vi "SMU Switch Handshaking - Debug.vi"(8 "error in":errorcluster, 11 "file path (use dialog)":path=path "/home/lvuser/jsontestfile.json") -> (0 "error out":errorcluster)   [LabVIEW 2019]
uses:
  labview-grpc-query-server/VIs/MeasurementServer_FourProbeRawData.ctl
  labview-grpc-query-server/VIs/MeasurementServer_ErrorOutData.ctl
  JSONCluster.ctl
  <instrlib>/niDCPower/nidcpower.llb/niDCPower Send Software Edge Trigger - Signal.ctl
  <instrlib>/niDCPower/nidcpower.llb/niDCPower Configure Software Edge Start Trigger.vi
  <instrlib>/niDCPower/nidcpower.llb/niDCPower Configure Software Edge Sequence Advance Trigger.vi
  SupportVIs.lvlib
  labview-grpc-query-server/VIs/labview-grpc-measurement-server.lvlib
panel:
  in  "Override Channel":bool=TRUE
  in  "Select Next Channel":i32=39
  out "Channels Connected":string[](array[string])=["[ab0->card2r0->c78]", "[ab1->card2r1->c79]", "[ab2->card2r2->c79]", "[ab3->card2r3->c78]"]
  in  "Override Settings":T1={"SMUResourceName"="SMU", "SMUChannels"="0", "SMUSourceMode"=1021, "SMUOutputFunction"=1007, "SMUSourceTransientResponse"=1038, "SMUCurrent"=1.0, "SMUCurrentLevelRange"=1.0, "SMUMeasurementSense"=1008, "SMUMeasurementApertureTime"=0.01, "SMUSourceAdvancedSourceDelay"=0.0001, "SMUVoltage"=6.0, "SMUSourceAdvancedSequenceLoopCount"=127, "SMUMeasurementAdvancedDCNoiseRejection"=1044, "SMUSequenceName"="MySequence", "SMUStep1_Source_DCCurrent_CurrentLevel"=1150009, "SMUStep2_Measurement_ApertureTime"=1150058, "SMUStep3_Source_Advanced_SourceDelay"=1150051, "SMUSequenceNumberOfSteps"=3, "ScanList"="ch0;ch1;ch2;ch3;ch4;ch5;ch6;ch7;ch8;ch9;ch10;ch11;ch12;ch13;ch14;ch15;ch16;ch17;ch18;ch19;ch20;ch21;ch22;ch23;ch24;ch25;ch26;ch27;ch28;ch29;ch30;ch31;ch32;ch33;ch34;ch35;ch36;ch37;ch38;ch39;ch40;ch41;ch42;ch43;ch44;ch45;ch46;ch47;ch48;ch49;ch50;ch51;ch52;ch53;ch54;ch55;ch56;ch57;ch58;ch59;ch60;ch61;ch62;ch63;ch64;ch65;ch66;ch67;ch68;ch69;ch70;ch71;ch72;ch73;ch74;ch75;ch76;ch77;ch78;ch79;ch80;ch81;ch82;ch83;ch84;ch85;ch86;ch87;ch88;ch89;ch90;ch91;ch92;ch93;ch94;ch95;ch96;ch97;ch98;ch99;ch100;ch101;ch102;ch103;ch104;ch105;ch106;ch107;ch108;ch109;ch110;ch111;ch112;ch113;ch114;ch115;ch116;ch117;ch118;ch119;ch120;ch121;ch122;ch123;ch124;ch125;ch126", "Switch1ResourceName"="2526_1", "Switch1Topology"="2526/2-Wire 79x1 Mux", "Switch1ScanList"="ch70:76->com", "Switch2ResourceName"="SwitchBlock1Dev1", "Switch2Topology"="Configured Topology", "Switch2ScanList"="[c2->card1r2->c26], [c3->card1r3->c27]; [c6->card1r2->c26], [c7->card1r3->c27]; [c10->card1r2->c26], [c11->card1r3->c27]; [c14->card1r2->c26], [c15->card1r3->c27]; [c18->card1r2->c26], [c19->card1r3->c27]; [c22->card1r2->c26], [c23->card1r3->c27]; [c30->card1r2->c26], [c31->card1r3->c27];", "DMMResourceName"="DMM", "DMMFunction"=0, "DMMResolution"=0.1, "DMMRange"=10.0, "DMMSampleCount"=0, "DMMApertureTimeUnit"=0, "DMMApertureTime"=0.01, "DMMNumberOfAverages"=1, "DMMAutoZero"=0, "DMMADCCalibration"=0, "DMMSettleTime"=0.0001, "DMMControlAction"=0, "DMMVoltageFaultUpperLimit"=0.0006, "ApplicationNumberOfWeldChannels"=127} {"DMMVoltageFaultUpperLimit" format="%#_6p"}
  in  "Override Settings?":bool=TRUE
  out "Configured Settings":T1={"SMUResourceName"="SMU", "SMUChannels"="0", "SMUSourceMode"=1021, "SMUOutputFunction"=1007, "SMUSourceTransientResponse"=1038, "SMUCurrent"=1.0, "SMUCurrentLevelRange"=1.0, "SMUMeasurementSense"=1008, "SMUMeasurementApertureTime"=0.01, "SMUSourceAdvancedSourceDelay"=0.0001, "SMUVoltage"=6.0, "SMUSourceAdvancedSequenceLoopCount"=127, "SMUMeasurementAdvancedDCNoiseRejection"=1044, "SMUSequenceName"="MySequence", "SMUStep1_Source_DCCurrent_CurrentLevel"=1150009, "SMUStep2_Measurement_ApertureTime"=1150058, "SMUStep3_Source_Advanced_SourceDelay"=1150051, "SMUSequenceNumberOfSteps"=3, "ScanList"="ch0;ch1;ch2;ch3;ch4;ch5;ch6;ch7;ch8;ch9;ch10;ch11;ch12;ch13;ch14;ch15;ch16;ch17;ch18;ch19;ch20;ch21;ch22;ch23;ch24;ch25;ch26;ch27;ch28;ch29;ch30;ch31;ch32;ch33;ch34;ch35;ch36;ch37;ch38;ch39;ch40;ch41;ch42;ch43;ch44;ch45;ch46;ch47;ch48;ch49;ch50;ch51;ch52;ch53;ch54;ch55;ch56;ch57;ch58;ch59;ch60;ch61;ch62;ch63;ch64;ch65;ch66;ch67;ch68;ch69;ch70;ch71;ch72;ch73;ch74;ch75;ch76;ch77;ch78;ch79;ch80;ch81;ch82;ch83;ch84;ch85;ch86;ch87;ch88;ch89;ch90;ch91;ch92;ch93;ch94;ch95;ch96;ch97;ch98;ch99;ch100;ch101;ch102;ch103;ch104;ch105;ch106;ch107;ch108;ch109;ch110;ch111;ch112;ch113;ch114;ch115;ch116;ch117;ch118;ch119;ch120;ch121;ch122;ch123;ch124;ch125;ch126", "Switch1ResourceName"="2526_1", "Switch1Topology"="2526/2-Wire 79x1 Mux", "Switch1ScanList"="ch70:76->com", "Switch2ResourceName"="SwitchBlock1Dev1", "Switch2Topology"="Configured Topology", "Switch2ScanList"="[c2->card1r2->c26], [c3->card1r3->c27]; [c6->card1r2->c26], [c7->card1r3->c27]; [c10->card1r2->c26], [c11->card1r3->c27]; [c14->card1r2->c26], [c15->card1r3->c27]; [c18->card1r2->c26], [c19->card1r3->c27]; [c22->card1r2->c26], [c23->card1r3->c27]; [c30->card1r2->c26], [c31->card1r3->c27];", "DMMResourceName"="DMM", "DMMFunction"=0, "DMMResolution"=0.1, "DMMRange"=10.0, "DMMSampleCount"=0, "DMMApertureTimeUnit"=0, "DMMApertureTime"=0.01, "DMMNumberOfAverages"=1, "DMMAutoZero"=0, "DMMADCCalibration"=0, "DMMSettleTime"=0.0001, "DMMControlAction"=0, "DMMVoltageFaultUpperLimit"=0.0006, "ApplicationNumberOfWeldChannels"=127} {"DMMVoltageFaultUpperLimit" format="%#_6p"}
  out "All Results":T2[](array[typedef])=[{"Positive Voltage"=0.4227098432914551, "Positive Current"=-8.493421060188494e-06, "Negative Voltage"=0.06989759298606142, "Negative Current"=-7.73956711993401e-06, "Impedance"=-468011.41635777906, "ErrorOutData"={"ErrorCode"=-3, "ErrorMessage"="SMU HI or LO lead disconnected\n- SMU in compliance\n- SMU Fault = True\rDMM HI SENSE or LO SENSE lead disconnected\n- DMM measures NaN, or \n- DMM overrange warning, or\n- DMM voltage > 50uV "}}, {"Positive Voltage"=0.00044270637570739045, "Positive Current"=0.9998336100314509, "Negative Voltage"=-0.0005552929370042879, "Negative Current"=-0.9996807598629482, "Impedance"=0.0004991208504114857, "ErrorOutData"={"ErrorCode"=0, "ErrorMessage"="\r"}}, {"Positive Voltage"=0.0004435264921852196, "Positive Current"=0.9998415883189853, "Negative Voltage"=-0.0005563935478104583, "Negative Current"=-0.9996805713994632, "Impedance"=0.000500079499062154, "ErrorOutData"={"ErrorCode"=0, "ErrorMessage"="\r"}}, {"Positive Voltage"=0.0004431847687781547, "Positive Current"=0.9998360600567567, "Negative Voltage"=-0.0005561418564061973, "Negative Current"=-0.999680791273529, "Impedance"=0.000499784047591045, "ErrorOutData"={"ErrorCode"=0, "ErrorMessage"="\r"}}, {"Positive Voltage"=0.0004426508664081714, "Positive Current"=0.9998373793011521, "Negative Voltage"=-0.0005564300544965975, "Negative Current"=-0.9996810739687567, "Impedance"=0.0004996607654562646, "ErrorOutData"={"ErrorCode"=0, "ErrorMessage"="\r"}}, {"Positive Voltage"=0.000442879495774044, "Positive Current"=0.9998407088227216, "Negative Voltage"=-0.0005564269589209733, "Negative Current"=-0.9996801630619121, "Impedance"=0.0004997729549845249, "ErrorOutData"={"ErrorCode"=0, "ErrorMessage"="\r"}}, {"Positive Voltage"=0.0004429170648054572, "Positive Current"=0.9998418396036319, "Negative Voltage"=-0.0005554367475981239, "Negative Current"=-0.9996802572936547, "Impedance"=0.0004992962138066661, "ErrorOutData"={"ErrorCode"=0, "ErrorMessage"="\r"}}, {"Positive Voltage"=0.0004437757493413744, "Positive Current"=0.9998415569084044, "Negative Voltage"=-0.0005568618872958528, "Negative Current"=-0.9996772418778936, "Impedance"=0.0005004392242996721, "ErrorOutData"={"ErrorCode"=0, "ErrorMessage"="\r"}}, {"Positive Voltage"=0.0004425981290562125, "Positive Current"=0.9998418710142127, "Negative Voltage"=-0.0005563588351510922, "Negative Current"=-0.9996784354799657, "Impedance"=0.0004995983091358584, "ErrorOutData"={"ErrorCode"=0, "ErrorMessage"="\r"}}, {"Positive Voltage"=0.0004431512451012525, "Positive Current"=0.999839829326458, "Negative Voltage"=-0.0005559987986000694, "Negative Current"=-0.9996786867646126, "Impedance"=0.0004996953194785092, "ErrorOutData"={"ErrorCode"=0, "ErrorMessage"="\r"}}, {"Positive Voltage"=0.0004428252458112706, "Positive Current"=0.9998417767824702, "Negative Voltage"=-0.0005563071531090114, "Negative Current"=-0.9996822361602478, "Impedance"=0.0004996851212853651, "ErrorOutData"={"ErrorCode"=0, "ErrorMessage"="\r"}}, {"Positive Voltage"=0.0004432269671022045, "Positive Current"=0.9998400177899429, "Negative Voltage"=-0.0005555003827833456, "Negative Current"=-0.9996774931625403, "Impedance"=0.0004994841727641584, "ErrorOutData"={"ErrorCode"=0, "ErrorMessage"="\r"}}, {"Positive Voltage"=0.00044334477486081486, "Positive Current"=0.9998417453718894, "Negative Voltage"=-0.0005564183194508279, "Negative Current"=-0.9996779329106722, "Impedance"=0.0005000016279761572, "ErrorOutData"={"ErrorCode"=0, "ErrorMessage"="\r"}}, {"Positive Voltage"=0.0004424807152799528, "Positive Current"=0.9998395466312303, "Negative Voltage"=-0.0005557886160507434, "Negative Current"=-0.9996787181751934, "Impedance"=0.0004992549199981127, "ErrorOutData"={"ErrorCode"=0, "ErrorMessage"="\r"}}, {"Positive Voltage"=0.00044335168362277214, "Positive Current"=0.9998386043138051, "Negative Voltage"=-0.0005557412185667331, "Negative Current"=-0.9996809797370141, "Impedance"=0.0004996664749666751, "ErrorOutData"={"ErrorCode"=0, "ErrorMessage"="\r"}}, {"Positive Voltage"=0.00044343080372150783, "Positive Current"=0.9998369395530203, "Negative Voltage"=-0.0005562687679712933, "Negative Current"=-0.9996811996110799, "Impedance"=0.0004999702438862225, "ErrorOutData"={"ErrorCode"=0, "ErrorMessage"="\r"}}, {"Positive Voltage"=0.0004416126595923773, "Positive Current"=0.9998378504598648, "Negative Voltage"=-0.0005565125515869184, "Negative Current"=-0.999679000870421, "Impedance"=0.0004991831954380576, "ErrorOutData"={"ErrorCode"=0, "ErrorMessage"="\r"}}, {"Positive Voltage"=0.0004425058457256834, "Positive Current"=0.9998383530291582, "Negative Voltage"=-0.0005561486666725616, "Negative Current"=-0.9996688552528084, "Impedance"=0.0004994503186894321, "ErrorOutData"={"ErrorCode"=0, "ErrorMessage"="\r"}}, {"Positive Voltage"=0.00044199289477433746, "Positive Current"=0.9998407402333024, "Negative Voltage"=-0.0005564866613180825, "Negative Current"=-0.9996799117772655, "Impedance"=0.0004993594615231526, "ErrorOutData"={"ErrorCode"=0, "ErrorMessage"="\r"}}, {"Positive Voltage"=0.00044318225010526666, "Positive Current"=0.9998403318957514, "Negative Voltage"=-0.0005570190932896488, "Negative Current"=-0.9996808855052717, "Impedance"=0.0005002204201138594, "ErrorOutData"={"ErrorCode"=0, "ErrorMessage"="\r"}}, {"Positive Voltage"=0.0004425723091413646, "Positive Current"=0.9998389184196134, "Negative Voltage"=-0.0005564301952045792, "Negative Current"=-0.9996751059583964, "Impedance"=0.0004996226543880852, "ErrorOutData"={"ErrorCode"=0, "ErrorMessage"="\r"}}, {"Positive Voltage"=0.0004422648410927191, "Positive Current"=0.9998419966565362, "Negative Voltage"=-0.0005559992699718129, "Negative Current"=-0.9996819220544393, "Impedance"=0.0004992508975376892, "ErrorOutData"={"ErrorCode"=0, "ErrorMessage"="\r"}}, {"Positive Voltage"=0.00044284054076900033, "Positive Current"=0.9998383530291582, "Negative Voltage"=-0.0005559332357154717, "Negative Current"=-0.9996781213741572, "Impedance"=0.0004995076506096407, "ErrorOutData"={"ErrorCode"=0, "ErrorMessage"="\r"}}, {"Positive Voltage"=0.00044220070639415055, "Positive Current"=0.9998387613667092, "Negative Voltage"=-0.0005564631279079567, "Negative Current"=-0.9996743835150368, "Impedance"=0.0004994534978969441, "ErrorOutData"={"ErrorCode"=0, "ErrorMessage"="\r"}}, {"Positive Voltage"=0.0004425694386985146, "Positive Current"=0.9998407402333024, "Negative Voltage"=-0.0005558320103926432, "Negative Current"=-0.9996787181751934, "Impedance"=0.0004993206967267169, "ErrorOutData"={"ErrorCode"=0, "ErrorMessage"="\r"}}, {"Positive Voltage"=0.00044327916976382933, "Positive Current"=0.9998404575380748, "Negative Voltage"=-0.0005567623363980099, "Negative Current"=-0.9996809169158525, "Impedance"=0.00050014044307726, "ErrorOutData"={"ErrorCode"=0, "ErrorMessage"="\r"}}, {"Positive Voltage"=0.000442306385124646, "Positive Current"=0.9998411171602725, "Negative Voltage"=-0.0005558222241524345, "Negative Current"=-0.9996798803666846, "Impedance"=0.0004991838597902116, "ErrorOutData"={"ErrorCode"=0, "ErrorMessage"="\r"}}, {"Positive Voltage"=0.00044307567787908264, "Positive Current"=0.9998385729032242, "Negative Voltage"=-0.0005561501018939907, "Negative Current"=-0.9996810425581757, "Impedance"=0.0004997329218710848, "ErrorOutData"={"ErrorCode"=0, "ErrorMessage"="\r"}}, {"Positive Voltage"=0.0004419110308699325, "Positive Current"=0.9998370651953438, "Negative Voltage"=-0.0005568956923887257, "Negative Current"=-0.9996802887042355, "Impedance"=0.0004995239082625241, "ErrorOutData"={"ErrorCode"=0, "ErrorMessage"="\r"}}, {"Positive Voltage"=0.00044257959781487293, "Positive Current"=0.9998401434322665, "Negative Voltage"=-0.0005564586393233032, "Negative Current"=-0.9996774303413787, "Impedance"=0.0004996396382016856, "ErrorOutData"={"ErrorCode"=0, "ErrorMessage"="\r"}}, {"Positive Voltage"=0.00044266013906423565, "Positive Current"=0.9998405203592365, "Negative Voltage"=-0.0005567629766193307, "Negative Current"=-0.9996879842965423, "Impedance"=0.0004998293914572717, "ErrorOutData"={"ErrorCode"=0, "ErrorMessage"="\r"}}, {"Positive Voltage"=0.0004422246267512286, "Positive Current"=0.9998426876893148, "Negative Voltage"=-0.0005563399873167974, "Negative Current"=-0.9996818906438585, "Impedance"=0.0004994010200667005, "ErrorOutData"={"ErrorCode"=0, "ErrorMessage"="\r"}}, {"Positive Voltage"=0.00044222253723768596, "Positive Current"=0.9998389184196134, "Negative Voltage"=-0.0005559288456264137, "Negative Current"=-0.9996776188048637, "Impedance"=0.0004991963628616098, "ErrorOutData"={"ErrorCode"=0, "ErrorMessage"="\r"}}, {"Positive Voltage"=0.00044335341433095643, "Positive Current"=0.9998379761021882, "Negative Voltage"=-0.0005566963584248685, "Negative Current"=-0.999682581676637, "Impedance"=0.0005001447816404218, "ErrorOutData"={"ErrorCode"=0, "ErrorMessage"="\r"}}, {"Positive Voltage"=0.00044284327753927097, "Positive Current"=0.999840426127494, "Negative Voltage"=-0.0005560568476783757, "Negative Current"=-0.9996789066386784, "Impedance"=0.000499570126104132, "ErrorOutData"={"ErrorCode"=0, "ErrorMessage"="\r"}}, {"Positive Voltage"=0.00044303544946679564, "Positive Current"=0.9998377562281222, "Negative Voltage"=-0.0005555104504395151, "Negative Current"=-0.9996565737156984, "Impedance"=0.0004993992155678514, "ErrorOutData"={"ErrorCode"=0, "ErrorMessage"="\r"}}, {"Positive Voltage"=0.0004430247275185058, "Positive Current"=0.9998403004851706, "Negative Voltage"=-0.0005556892058608842, "Negative Current"=-0.9996790636915827, "Impedance"=0.000499476999959229, "ErrorOutData"={"ErrorCode"=0, "ErrorMessage"="\r"}}, {"Positive Voltage"=0.0004431882231591376, "Positive Current"=0.9998384786714817, "Negative Voltage"=-0.0005559463074870784, "Negative Current"=-0.9996799745984271, "Impedance"=0.0004996875767824414, "ErrorOutData"={"ErrorCode"=0, "ErrorMessage"="\r"}}, {"Positive Voltage"=0.0004431953218768679, "Positive Current"=0.9998368767318586, "Negative Voltage"=-0.0005563412396178422, "Negative Current"=-0.9996809797370141, "Impedance"=0.0004998887898205026, "ErrorOutData"={"ErrorCode"=0, "ErrorMessage"="\r"}}, {"Positive Voltage"=0.00044275691801481633, "Positive Current"=0.9998376934069605, "Negative Voltage"=-0.0005565454420779015, "Negative Current"=-0.9996735982505158, "Impedance"=0.0004997733017373237, "ErrorOutData"={"ErrorCode"=0, "ErrorMessage"="\r"}}, {"Positive Voltage"=0.00044314802288844546, "Positive Current"=0.9998382902079966, "Negative Voltage"=-0.0005562527554028524, "Negative Current"=-0.9996796919031994, "Impedance"=0.0004998208504412039, "ErrorOutData"={"ErrorCode"=0, "ErrorMessage"="\r"}}, {"Positive Voltage"=0.0004420522031890927, "Positive Current"=0.9998410229285299, "Negative Voltage"=-0.0005573198777091121, "Negative Current"=-0.9996810111475949, "Impedance"=0.0004998054854444067, "ErrorOutData"={"ErrorCode"=0, "ErrorMessage"="\r"}}, {"Positive Voltage"=0.00044142678434708, "Positive Current"=0.9998407716438832, "Negative Voltage"=-0.0005555250137157432, "Negative Current"=-0.9996751373689772, "Impedance"=0.0004985965820872151, "ErrorOutData"={"ErrorCode"=0, "ErrorMessage"="\r"}}, {"Positive Voltage"=0.000443285860428411, "Positive Current"=0.9998395466312303, "Negative Voltage"=-0.0005562909083723878, "Negative Current"=-0.9996787181751934, "Impedance"=0.0004999087962307609, "ErrorOutData"={"ErrorCode"=0, "ErrorMessage"="\r"}}, {"Positive Voltage"=0.0004429727148126581, "Positive Current"=0.9998380389233499, "Negative Voltage"=-0.0005558561207054957, "Negative Current"=-0.9996800688301695, "Impedance"=0.000499534778727435, "ErrorOutData"={"ErrorCode"=0, "ErrorMessage"="\r"}}, {"Positive Voltage"=0.00044351776829028403, "Positive Current"=0.9998382902079966, "Negative Voltage"=-0.0005558105664960561, "Negative Current"=-0.9996829271930263, "Impedance"=0.0004997838112892179, "ErrorOutData"={"ErrorCode"=0, "ErrorMessage"="\r"}}, {"Positive Voltage"=0.00044180997439667607, "Positive Current"=0.9998401120216855, "Negative Voltage"=-0.000557451756266006, "Negative Current"=-0.9996774303413787, "Impedance"=0.0004997514197758612, "ErrorOutData"={"ErrorCode"=0, "ErrorMessage"="\r"}}, {"Positive Voltage"=0.00044238172017864306, "Positive Current"=0.9998386043138051, "Negative Voltage"=-0.0005569053801333431, "Negative Current"=-0.9996742578727136, "Impedance"=0.0004997652774382456, "ErrorOutData"={"ErrorCode"=0, "ErrorMessage"="\r"}}, {"Positive Voltage"=0.0004427133055755449, "Positive Current"=0.9998418710142127, "Negative Voltage"=-0.0005560911241429957, "Negative Current"=-0.9996782156058999, "Impedance"=0.0004995220785237866, "ErrorOutData"={"ErrorCode"=0, "ErrorMessage"="\r"}}, {"Positive Voltage"=0.0004414873591336821, "Positive Current"=0.9998379446916074, "Negative Voltage"=-0.0005556362926239444, "Negative Current"=-0.9996797547243612, "Impedance"=0.000498682083208802, "ErrorOutData"={"ErrorCode"=0, "ErrorMessage"="\r"}}, {"Positive Voltage"=0.0004430884963763173, "Positive Current"=0.999840426127494, "Negative Voltage"=-0.0005560188072752255, "Negative Current"=-0.9996811996110799, "Impedance"=0.0004996731672169323, "ErrorOutData"={"ErrorCode"=0, "ErrorMessage"="\r"}}, {"Positive Voltage"=0.00044224104033742503, "Positive Current"=0.9998412113920151, "Negative Voltage"=-0.0005563428929366435, "Negative Current"=-0.9996808540946909, "Impedance"=0.0004994113095876249, "ErrorOutData"={"ErrorCode"=0, "ErrorMessage"="\r"}}, {"Positive Voltage"=0.0004429970643290835, "Positive Current"=0.9998384786714817, "Negative Voltage"=-0.000556510075126418, "Negative Current"=-0.9996776502154447, "Impedance"=0.0004998745071448354, "ErrorOutData"={"ErrorCode"=0, "ErrorMessage"="\r"}}, {"Positive Voltage"=0.00044266864486179787, "Positive Current"=0.9998386043138051, "Negative Voltage"=-0.0005569831564708411, "Negative Current"=-0.9996800374195887, "Impedance"=0.000499946227291002, "ErrorOutData"={"ErrorCode"=0, "ErrorMessage"="\r"}}, {"Positive Voltage"=0.0004427809439028817, "Positive Current"=0.9998398607370388, "Negative Voltage"=-0.0005559008939856245, "Negative Current"=-0.9996806970417864, "Impedance"=0.0004994606502060152, "ErrorOutData"={"ErrorCode"=0, "ErrorMessage"="\r"}}, {"Positive Voltage"=0.00044351095098851617, "Positive Current"=0.9998402690745898, "Negative Voltage"=-0.0005555750424390234, "Negative Current"=-0.9996839637421944, "Impedance"=0.0004996618580711573, "ErrorOutData"={"ErrorCode"=0, "ErrorMessage"="\r"}}, {"Positive Voltage"=0.0004428245211651586, "Positive Current"=0.9998405203592365, "Negative Voltage"=-0.0005560609563514788, "Negative Current"=-0.9996781841953188, "Impedance"=0.0004995629574463847, "ErrorOutData"={"ErrorCode"=0, "ErrorMessage"="\r"}}, {"Positive Voltage"=0.00044282480961652413, "Positive Current"=0.9998400806111047, "Negative Voltage"=-0.000555894519914007, "Negative Current"=-0.9996828957824455, "Impedance"=0.0004994787963536564, "ErrorOutData"={"ErrorCode"=0, "ErrorMessage"="\r"}}, {"Positive Voltage"=0.00044260601573864906, "Positive Current"=0.9998393267571645, "Negative Voltage"=-0.000556537344333492, "Negative Current"=-0.9996795034397143, "Impedance"=0.0004996918983622485, "ErrorOutData"={"ErrorCode"=0, "ErrorMessage"="\r"}}, {"Positive Voltage"=0.00044254660179290423, "Positive Current"=0.9998405831803983, "Negative Voltage"=-0.000556063974537708, "Negative Current"=-0.9996802572936547, "Impedance"=0.00049942494027412, "ErrorOutData"={"ErrorCode"=0, "ErrorMessage"="\r"}}, {"Positive Voltage"=0.00044281629678356534, "Positive Current"=0.9998393267571645, "Negative Voltage"=-0.0005562237976999881, "Negative Current"=-0.9996801002407505, "Impedance"=0.0004996401040141508, "ErrorOutData"={"ErrorCode"=0, "ErrorMessage"="\r"}}, {"Positive Voltage"=0.0004432513095832306, "Positive Current"=0.9998374421223138, "Negative Voltage"=-0.0005564357039221052, "Negative Current"=-0.9996799117772655, "Impedance"=0.0004999641596286653, "ErrorOutData"={"ErrorCode"=0, "ErrorMessage"="\r"}}, {"Positive Voltage"=0.00044258595078029803, "Positive Current"=0.9998409286967875, "Negative Voltage"=-0.0005558095111861886, "Negative Current"=-0.9996796604926186, "Impedance"=0.0004993174200677926, "ErrorOutData"={"ErrorCode"=0, "ErrorMessage"="\r"}}, {"Positive Voltage"=0.00044370010472981504, "Positive Current"=0.9998396408629728, "Negative Voltage"=-0.0005551230180442423, "Negative Current"=-0.9996802258830739, "Impedance"=0.0004995314822250351, "ErrorOutData"={"ErrorCode"=0, "ErrorMessage"="\r"}}, {"Positive Voltage"=0.0004421424532892677, "Positive Current"=0.9998386043138051, "Negative Voltage"=-0.0005560646288298306, "Negative Current"=-0.9996828957824455, "Impedance"=0.0004992229801335208, "ErrorOutData"={"ErrorCode"=0, "ErrorMessage"="\r"}}, {"Positive Voltage"=0.0004429717157859826, "Positive Current"=0.9998399549687813, "Negative Voltage"=-0.000554845260486166, "Negative Current"=-0.9996752630113004, "Impedance"=0.0004990294483880684, "ErrorOutData"={"ErrorCode"=0, "ErrorMessage"="\r"}}, {"Positive Voltage"=0.0004434583543445421, "Positive Current"=0.9998400806111047, "Negative Voltage"=-0.0005564016807318582, "Negative Current"=-0.9996788124069358, "Impedance"=0.0005000503063850666, "ErrorOutData"={"ErrorCode"=0, "ErrorMessage"="\r"}}, {"Positive Voltage"=0.00044290748259182754, "Positive Current"=0.9998385100820625, "Negative Voltage"=-0.0005550344001566628, "Negative Current"=-0.9996828015507031, "Impedance"=0.0004990903957575691, "ErrorOutData"={"ErrorCode"=0, "ErrorMessage"="\r"}}, {"Positive Voltage"=0.00044336150503997346, "Positive Current"=0.9998409601073683, "Negative Voltage"=-0.000556003906299844, "Negative Current"=-0.9996812310216607, "Impedance"=0.0004998021106109987, "ErrorOutData"={"ErrorCode"=0, "ErrorMessage"="\r"}}, {"Positive Voltage"=0.00044301018534848176, "Positive Current"=0.9998403318957514, "Negative Voltage"=-0.0005556932371445914, "Negative Current"=-0.9996803829359779, "Impedance"=0.0004994714058649398, "ErrorOutData"={"ErrorCode"=0, "ErrorMessage"="\r"}}, {"Positive Voltage"=0.0004430160036235707, "Positive Current"=0.99983841585032, "Negative Voltage"=-0.0005551907900441595, "Negative Current"=-0.9996821733390862, "Impedance"=0.0004992230633005871, "ErrorOutData"={"ErrorCode"=0, "ErrorMessage"="\r"}}, {"Positive Voltage"=0.00044397347923422236, "Positive Current"=0.9998403004851706, "Negative Voltage"=-0.0005554320690576878, "Negative Current"=-0.9996791265127443, "Impedance"=0.0004998228748356905, "ErrorOutData"={"ErrorCode"=0, "ErrorMessage"="\r"}}, {"Positive Voltage"=0.0004427937975771129, "Positive Current"=0.9998398607370388, "Negative Voltage"=-0.0005560462101548804, "Negative Current"=-0.9996791893339061, "Impedance"=0.0004995401307612215, "ErrorOutData"={"ErrorCode"=0, "ErrorMessage"="\r"}}, {"Positive Voltage"=0.0004433314005670486, "Positive Current"=0.9998418081930511, "Negative Voltage"=-0.0005552790772679779, "Negative Current"=-0.9996795348502954, "Impedance"=0.0004994247654866759, "ErrorOutData"={"ErrorCode"=0, "ErrorMessage"="\r"}}, {"Positive Voltage"=0.00044341707062238586, "Positive Current"=0.9998393581677453, "Negative Voltage"=-0.0005556148205857652, "Negative Current"=-0.9996809797370141, "Impedance"=0.0004996357737751287, "ErrorOutData"={"ErrorCode"=0, "ErrorMessage"="\r"}}, {"Positive Voltage"=0.0004425868794529835, "Positive Current"=0.9998395780418111, "Negative Voltage"=-0.0005556132587271592, "Negative Current"=-0.9996740065880667, "Impedance"=0.0004992214835914284, "ErrorOutData"={"ErrorCode"=0, "ErrorMessage"="\r"}}, {"Positive Voltage"=0.0004435337456817334, "Positive Current"=0.9998420280671171, "Negative Voltage"=-0.0005550171001101737, "Negative Current"=-0.9996788124069358, "Impedance"=0.0004993950678479388, "ErrorOutData"={"ErrorCode"=0, "ErrorMessage"="\r"}}, {"Positive Voltage"=0.0004429351035688524, "Positive Current"=0.9998386357243859, "Negative Voltage"=-0.000554562233414135, "Negative Current"=-0.9996781841953188, "Impedance"=0.0004988691903192113, "ErrorOutData"={"ErrorCode"=0, "ErrorMessage"="\r"}}, {"Positive Voltage"=0.0004439495518417443, "Positive Current"=0.9998382273868349, "Negative Voltage"=-0.0005553659996243591, "Negative Current"=-0.9996779015000914, "Impedance"=0.0004997786899685545, "ErrorOutData"={"ErrorCode"=0, "ErrorMessage"="\r"}}, {"Positive Voltage"=0.00044354244847046975, "Positive Current"=0.9998349606864272, "Negative Voltage"=-0.0005560542656868961, "Negative Current"=-0.999678152784738, "Impedance"=0.0004999200592498544, "ErrorOutData"={"ErrorCode"=0, "ErrorMessage"="\r"}}, {"Positive Voltage"=0.0004426065222873858, "Positive Current"=0.9998414312660809, "Negative Voltage"=-0.0005557233556883142, "Negative Current"=-0.9996766764874385, "Impedance"=0.0004992852398307783, "ErrorOutData"={"ErrorCode"=0, "ErrorMessage"="\r"}}, {"Positive Voltage"=0.00044288011488916983, "Positive Current"=0.9998413684449193, "Negative Voltage"=-0.0005557669892337818, "Negative Current"=-0.999679786134942, "Impedance"=0.0004994431300892072, "ErrorOutData"={"ErrorCode"=0, "ErrorMessage"="\r"}}, {"Positive Voltage"=0.0004428762032072458, "Positive Current"=0.9998377248175414, "Negative Voltage"=-0.0005548895553591558, "Negative Current"=-0.999676959182666, "Impedance"=0.0004990039665876733, "ErrorOutData"={"ErrorCode"=0, "ErrorMessage"="\r"}}, {"Positive Voltage"=0.00044407517592880336, "Positive Current"=0.999837787638703, "Negative Voltage"=-0.0005548592187180599, "Negative Current"=-0.9996804771677206, "Impedance"=0.0004995875317715949, "ErrorOutData"={"ErrorCode"=0, "ErrorMessage"="\r"}}, {"Positive Voltage"=0.000442873438295384, "Positive Current"=0.9998397665052963, "Negative Voltage"=-0.0005559368941230299, "Negative Current"=-0.9996825502660562, "Impedance"=0.0004995244734408377, "ErrorOutData"={"ErrorCode"=0, "ErrorMessage"="\r"}}, {"Positive Voltage"=0.00044300414897601896, "Positive Current"=0.9998385100820625, "Negative Voltage"=-0.0005553567410390924, "Negative Current"=-0.99967859253287, "Impedance"=0.0004993010005813268, "ErrorOutData"={"ErrorCode"=0, "ErrorMessage"="\r"}}, {"Positive Voltage"=0.00044446186960717495, "Positive Current"=0.9998381959762541, "Negative Voltage"=-0.0005549508266502684, "Negative Current"=-0.9996785297117083, "Impedance"=0.0004998271249336918, "ErrorOutData"={"ErrorCode"=0, "ErrorMessage"="\r"}}, {"Positive Voltage"=0.00044342652619882645, "Positive Current"=0.9998413998555001, "Negative Voltage"=-0.0005558535176078165, "Negative Current"=-0.9996788438175166, "Impedance"=0.0004997599033911337, "ErrorOutData"={"ErrorCode"=0, "ErrorMessage"="\r"}}, {"Positive Voltage"=0.0004433281853896422, "Positive Current"=0.9998417139613086, "Negative Voltage"=-0.0005547129879469202, "Negative Current"=-0.9996754200642048, "Impedance"=0.0004991410957940947, "ErrorOutData"={"ErrorCode"=0, "ErrorMessage"="\r"}}, {"Positive Voltage"=0.0004441760213400837, "Positive Current"=0.9998393895783262, "Negative Voltage"=-0.0005557373279910032, "Negative Current"=-0.9996753886536238, "Impedance"=0.0005000779990309699, "ErrorOutData"={"ErrorCode"=0, "ErrorMessage"="\r"}}, {"Positive Voltage"=0.0004441705266933572, "Positive Current"=0.9998400177899429, "Negative Voltage"=-0.0005539599117875031, "Negative Current"=-0.9996783412482233, "Impedance"=0.0004991854333165481, "ErrorOutData"={"ErrorCode"=0, "ErrorMessage"="\r"}}, {"Positive Voltage"=0.0004443011881261959, "Positive Current"=0.9998402690745898, "Negative Voltage"=-0.0005546106721372168, "Negative Current"=-0.9996799745984271, "Impedance"=0.000499575767449327, "ErrorOutData"={"ErrorCode"=0, "ErrorMessage"="\r"}}, {"Positive Voltage"=0.000443970418835595, "Positive Current"=0.9998430646162849, "Negative Voltage"=-0.0005559718600567603, "Negative Current"=-0.9996837124575475, "Impedance"=0.0005000894663464827, "ErrorOutData"={"ErrorCode"=0, "ErrorMessage"="\r"}}, {"Positive Voltage"=0.00044269900964449057, "Positive Current"=0.9998405831803983, "Negative Voltage"=-0.0005546125787303834, "Negative Current"=-0.999673535429354, "Impedance"=0.0004987769674106114, "ErrorOutData"={"ErrorCode"=0, "ErrorMessage"="\r"}}, {"Positive Voltage"=0.00044476273845142405, "Positive Current"=0.999839201114841, "Negative Voltage"=-0.0005547441406943128, "Negative Current"=-0.9996797233137802, "Impedance"=0.0004998736780805183, "ErrorOutData"={"ErrorCode"=0, "ErrorMessage"="\r"}}, {"Positive Voltage"=0.0004437515686745285, "Positive Current"=0.9998401434322665, "Negative Voltage"=-0.0005555780395190644, "Negative Current"=-0.999680791273529, "Impedance"=0.0004997845188055667, "ErrorOutData"={"ErrorCode"=0, "ErrorMessage"="\r"}}, {"Positive Voltage"=0.00044478751712719494, "Positive Current"=0.9998395780418111, "Negative Voltage"=-0.0005546307652371631, "Negative Current"=-0.9996826444977989, "Impedance"=0.0004998285445885109, "ErrorOutData"={"ErrorCode"=0, "ErrorMessage"="\r"}}, {"Positive Voltage"=0.0004436276471540641, "Positive Current"=0.999839829326458, "Negative Voltage"=-0.0005545804621333089, "Negative Current"=-0.9996774617519595, "Impedance"=0.0004992245447144898, "ErrorOutData"={"ErrorCode"=0, "ErrorMessage"="\r"}}, {"Positive Voltage"=0.0004442093198842178, "Positive Current"=0.9998427190998956, "Negative Voltage"=-0.000554744802021834, "Negative Current"=-0.9996790322810019, "Impedance"=0.0004995965266275099, "ErrorOutData"={"ErrorCode"=0, "ErrorMessage"="\r"}}, {"Positive Voltage"=0.00044512598314445673, "Positive Current"=0.9998256945650782, "Negative Voltage"=-0.0005556313889507473, "Negative Current"=-0.9996786867646126, "Impedance"=0.0005005027152927218, "ErrorOutData"={"ErrorCode"=0, "ErrorMessage"="\r"}}, {"Positive Voltage"=0.00044217321205431066, "Positive Current"=0.9998455460521715, "Negative Voltage"=-0.000555220317614351, "Negative Current"=-0.9996705514241739, "Impedance"=0.0004988174543468315, "ErrorOutData"={"ErrorCode"=0, "ErrorMessage"="\r"}}, {"Positive Voltage"=-5.4936250649797755e-05, "Positive Current"=-8.399189317657985e-06, "Negative Voltage"=-5.6232501835270916e-05, "Negative Current"=-7.770977700782139e-06, "Impedance"=-2.0633989417762395, "ErrorOutData"={"ErrorCode"=-1, "ErrorMessage"="SMU HI or LO lead disconnected\n- SMU in compliance\n- SMU Fault = True\r"}}, {"Positive Voltage"=-5.5786872618300966e-05, "Positive Current"=-8.556242221877813e-06, "Negative Voltage"=-5.625998210431502e-05, "Negative Current"=-7.67674595824816e-06, "Impedance"=-0.5379323432956326, "ErrorOutData"={"ErrorCode"=-1, "ErrorMessage"="SMU HI or LO lead disconnected\n- SMU in compliance\n- SMU Fault = True\r"}}, {"Positive Voltage"=-5.679127434122135e-05, "Positive Current"=-8.493421060188494e-06, "Negative Voltage"=-5.500922180968423e-05, "Negative Current"=-7.896620024153839e-06, "Impedance"=2.9860077713297404, "ErrorOutData"={"ErrorCode"=-1, "ErrorMessage"="SMU HI or LO lead disconnected\n- SMU in compliance\n- SMU Fault = True\r"}}, {"Positive Voltage"=-5.585377222872932e-05, "Positive Current"=-8.493421060188494e-06, "Negative Voltage"=-5.6387027341996994e-05, "Negative Current"=-7.6453353774035e-06, "Impedance"=-0.628775044894683, "ErrorOutData"={"ErrorCode"=-1, "ErrorMessage"="SMU HI or LO lead disconnected\n- SMU in compliance\n- SMU Fault = True\r"}}, {"Positive Voltage"=-5.5937845248460853e-05, "Positive Current"=-8.367778736813325e-06, "Negative Voltage"=-5.589400767641558e-05, "Negative Current"=-7.896620024153839e-06, "Impedance"=0.09304204903233429, "ErrorOutData"={"ErrorCode"=-1, "ErrorMessage"="SMU HI or LO lead disconnected\n- SMU in compliance\n- SMU Fault = True\r"}}, {"Positive Voltage"=-5.5435609210005034e-05, "Positive Current"=-8.367778736813325e-06, "Negative Voltage"=-5.577877487389006e-05, "Negative Current"=-7.331229568967312e-06, "Impedance"=-0.3310654955212006, "ErrorOutData"={"ErrorCode"=-1, "ErrorMessage"="SMU HI or LO lead disconnected\n- SMU in compliance\n- SMU Fault = True\r"}}, {"Positive Voltage"=-5.546069744334024e-05, "Positive Current"=-7.896620024153839e-06, "Negative Voltage"=-5.547551399393069e-05, "Negative Current"=-7.67674595824816e-06, "Impedance"=-0.06738653114646379, "ErrorOutData"={"ErrorCode"=-1, "ErrorMessage"="SMU HI or LO lead disconnected\n- SMU in compliance\n- SMU Fault = True\r"}}, {"Positive Voltage"=-5.6055399732703e-05, "Positive Current"=-7.959441185843158e-06, "Negative Voltage"=-5.459200856984353e-05, "Negative Current"=-7.551103634872991e-06, "Impedance"=3.5837780762082767, "ErrorOutData"={"ErrorCode"=-1, "ErrorMessage"="SMU HI or LO lead disconnected\n- SMU in compliance\n- SMU Fault = True\r"}}, {"Positive Voltage"=-5.516195328962939e-05, "Positive Current"=-8.336368155968665e-06, "Negative Voltage"=-5.677059026774827e-05, "Negative Current"=-7.6453353774035e-06, "Impedance"=-2.327873623388742, "ErrorOutData"={"ErrorCode"=-1, "ErrorMessage"="SMU HI or LO lead disconnected\n- SMU in compliance\n- SMU Fault = True\r"}}, {"Positive Voltage"=-5.575575504790172e-05, "Positive Current"=-8.085083509218327e-06, "Negative Voltage"=-5.57937039908661e-05, "Negative Current"=-7.551103634872991e-06, "Impedance"=-0.07106811471295137, "ErrorOutData"={"ErrorCode"=-1, "ErrorMessage"="SMU HI or LO lead disconnected\n- SMU in compliance\n- SMU Fault = True\r"}}, {"Positive Voltage"=-5.548912749126724e-05, "Positive Current"=-8.179315251752306e-06, "Negative Voltage"=-5.56106851176201e-05, "Negative Current"=-7.770977700782139e-06, "Impedance"=-0.2976890713676665, "ErrorOutData"={"ErrorCode"=-1, "ErrorMessage"="SMU HI or LO lead disconnected\n- SMU in compliance\n- SMU Fault = True\r"}}, {"Positive Voltage"=-5.496817729109712e-05, "Positive Current"=-8.587652802719004e-06, "Negative Voltage"=-5.679008535876615e-05, "Negative Current"=-7.770977700782139e-06, "Impedance"=-2.230884795371018, "ErrorOutData"={"ErrorCode"=-1, "ErrorMessage"="SMU HI or LO lead disconnected\n- SMU in compliance\n- SMU Fault = True\r"}}, {"Positive Voltage"=-5.581537302021944e-05, "Positive Current"=-8.147904670907646e-06, "Negative Voltage"=-5.514245116321133e-05, "Negative Current"=-7.582514215717651e-06, "Impedance"=1.1901896306013517, "ErrorOutData"={"ErrorCode"=-1, "ErrorMessage"="SMU HI or LO lead disconnected\n- SMU in compliance\n- SMU Fault = True\r"}}, {"Positive Voltage"=-5.5946871665558414e-05, "Positive Current"=-8.022262347532477e-06, "Negative Voltage"=-5.701114463516627e-05, "Negative Current"=-7.331229568967312e-06, "Impedance"=-1.5401193729444707, "ErrorOutData"={"ErrorCode"=-1, "ErrorMessage"="SMU HI or LO lead disconnected\n- SMU in compliance\n- SMU Fault = True\r"}}, {"Positive Voltage"=-5.535246486296016e-05, "Positive Current"=-8.242136413438156e-06, "Negative Voltage"=-5.564194339600249e-05, "Negative Current"=-8.116494090062987e-06, "Impedance"=-2.303989016328083, "ErrorOutData"={"ErrorCode"=-1, "ErrorMessage"="SMU HI or LO lead disconnected\n- SMU in compliance\n- SMU Fault = True\r"}}, {"Positive Voltage"=-5.546840824079897e-05, "Positive Current"=-8.210725832596966e-06, "Negative Voltage"=-5.535606698731934e-05, "Negative Current"=-7.2369978264333334e-06, "Impedance"=0.11537231420737543, "ErrorOutData"={"ErrorCode"=-1, "ErrorMessage"="SMU HI or LO lead disconnected\n- SMU in compliance\n- SMU Fault = True\r"}}, {"Positive Voltage"=-5.5370285528983344e-05, "Positive Current"=-8.210725832596966e-06, "Negative Voltage"=-5.6517266650889724e-05, "Negative Current"=-7.582514215717651e-06, "Impedance"=-1.8257878254529718, "ErrorOutData"={"ErrorCode"=-1, "ErrorMessage"="SMU HI or LO lead disconnected\n- SMU in compliance\n- SMU Fault = True\r"}}, {"Positive Voltage"=-5.679598102324659e-05, "Positive Current"=-8.430599898502644e-06, "Negative Voltage"=-5.5887478826012276e-05, "Negative Current"=-7.394050730653162e-06, "Impedance"=0.8764680204405331, "ErrorOutData"={"ErrorCode"=-1, "ErrorMessage"="SMU HI or LO lead disconnected\n- SMU in compliance\n- SMU Fault = True\r"}}, {"Positive Voltage"=-5.562586750896585e-05, "Positive Current"=-7.928030604998498e-06, "Negative Voltage"=-5.558539285770984e-05, "Negative Current"=-7.582514215717651e-06, "Impedance"=0.11714249312529738, "ErrorOutData"={"ErrorCode"=-1, "ErrorMessage"="SMU HI or LO lead disconnected\n- SMU in compliance\n- SMU Fault = True\r"}}, {"Positive Voltage"=-5.638317897866737e-05, "Positive Current"=-8.242136413438156e-06, "Negative Voltage"=-5.589961488953034e-05, "Negative Current"=-7.928030604998498e-06, "Impedance"=1.5394942600366655, "ErrorOutData"={"ErrorCode"=-1, "ErrorMessage"="SMU HI or LO lead disconnected\n- SMU in compliance\n- SMU Fault = True\r"}}, {"Positive Voltage"=-5.674339141466974e-05, "Positive Current"=-7.990851766687818e-06, "Negative Voltage"=-5.492464927661395e-05, "Negative Current"=-7.519693054028331e-06, "Impedance"=3.860147523941097, "ErrorOutData"={"ErrorCode"=-1, "ErrorMessage"="SMU HI or LO lead disconnected\n- SMU in compliance\n- SMU Fault = True\r"}}, {"Positive Voltage"=-5.536608539569625e-05, "Positive Current"=-8.116494090062987e-06, "Negative Voltage"=-5.6022157471762884e-05, "Negative Current"=-7.70815653909282e-06, "Impedance"=-1.606690529704838, "ErrorOutData"={"ErrorCode"=-1, "ErrorMessage"="SMU HI or LO lead disconnected\n- SMU in compliance\n- SMU Fault = True\r"}}, {"Positive Voltage"=-5.619925957433174e-05, "Positive Current"=-8.053672928373667e-06, "Negative Voltage"=-5.55028887319867e-05, "Negative Current"=-7.3626401498085026e-06, "Impedance"=1.0077247620452379, "ErrorOutData"={"ErrorCode"=-1, "ErrorMessage"="SMU HI or LO lead disconnected\n- SMU in compliance\n- SMU Fault = True\r"}}, {"Positive Voltage"=-5.6131149875250484e-05, "Positive Current"=-8.587652802719004e-06, "Negative Voltage"=-5.562473480970491e-05, "Negative Current"=-7.582514215717651e-06, "Impedance"=0.5038261112394141, "ErrorOutData"={"ErrorCode"=-1, "ErrorMessage"="SMU HI or LO lead disconnected\n- SMU in compliance\n- SMU Fault = True\r"}}, {"Positive Voltage"=-5.5605099010702733e-05, "Positive Current"=-8.085083509218327e-06, "Negative Voltage"=-5.631928348367192e-05, "Negative Current"=-7.61392479656231e-06, "Impedance"=-1.5158044492973206, "ErrorOutData"={"ErrorCode"=-1, "ErrorMessage"="SMU HI or LO lead disconnected\n- SMU in compliance\n- SMU Fault = True\r"}}, {"Positive Voltage"=-5.6192266387585296e-05, "Positive Current"=-8.430599898502644e-06, "Negative Voltage"=-5.535022760603262e-05, "Negative Current"=-7.488282473183672e-06, "Impedance"=0.8935829466038484, "ErrorOutData"={"ErrorCode"=-1, "ErrorMessage"="SMU HI or LO lead disconnected\n- SMU in compliance\n- SMU Fault = True\r"}}]
  in  "Default Results":T2[](array[typedef])
  out "Channel Index":i32=39
  out "Result":T2={"Positive Voltage"=-5.5605099010702733e-05, "Positive Current"=-8.085083509218327e-06, "Negative Voltage"=-5.631928348367192e-05, "Negative Current"=-7.61392479656231e-06, "Impedance"=-1.5158044492973206, "ErrorOutData"={"ErrorCode"=-1, "ErrorMessage"="SMU HI or LO lead disconnected\n- SMU in compliance\n- SMU Fault = True\r"}}
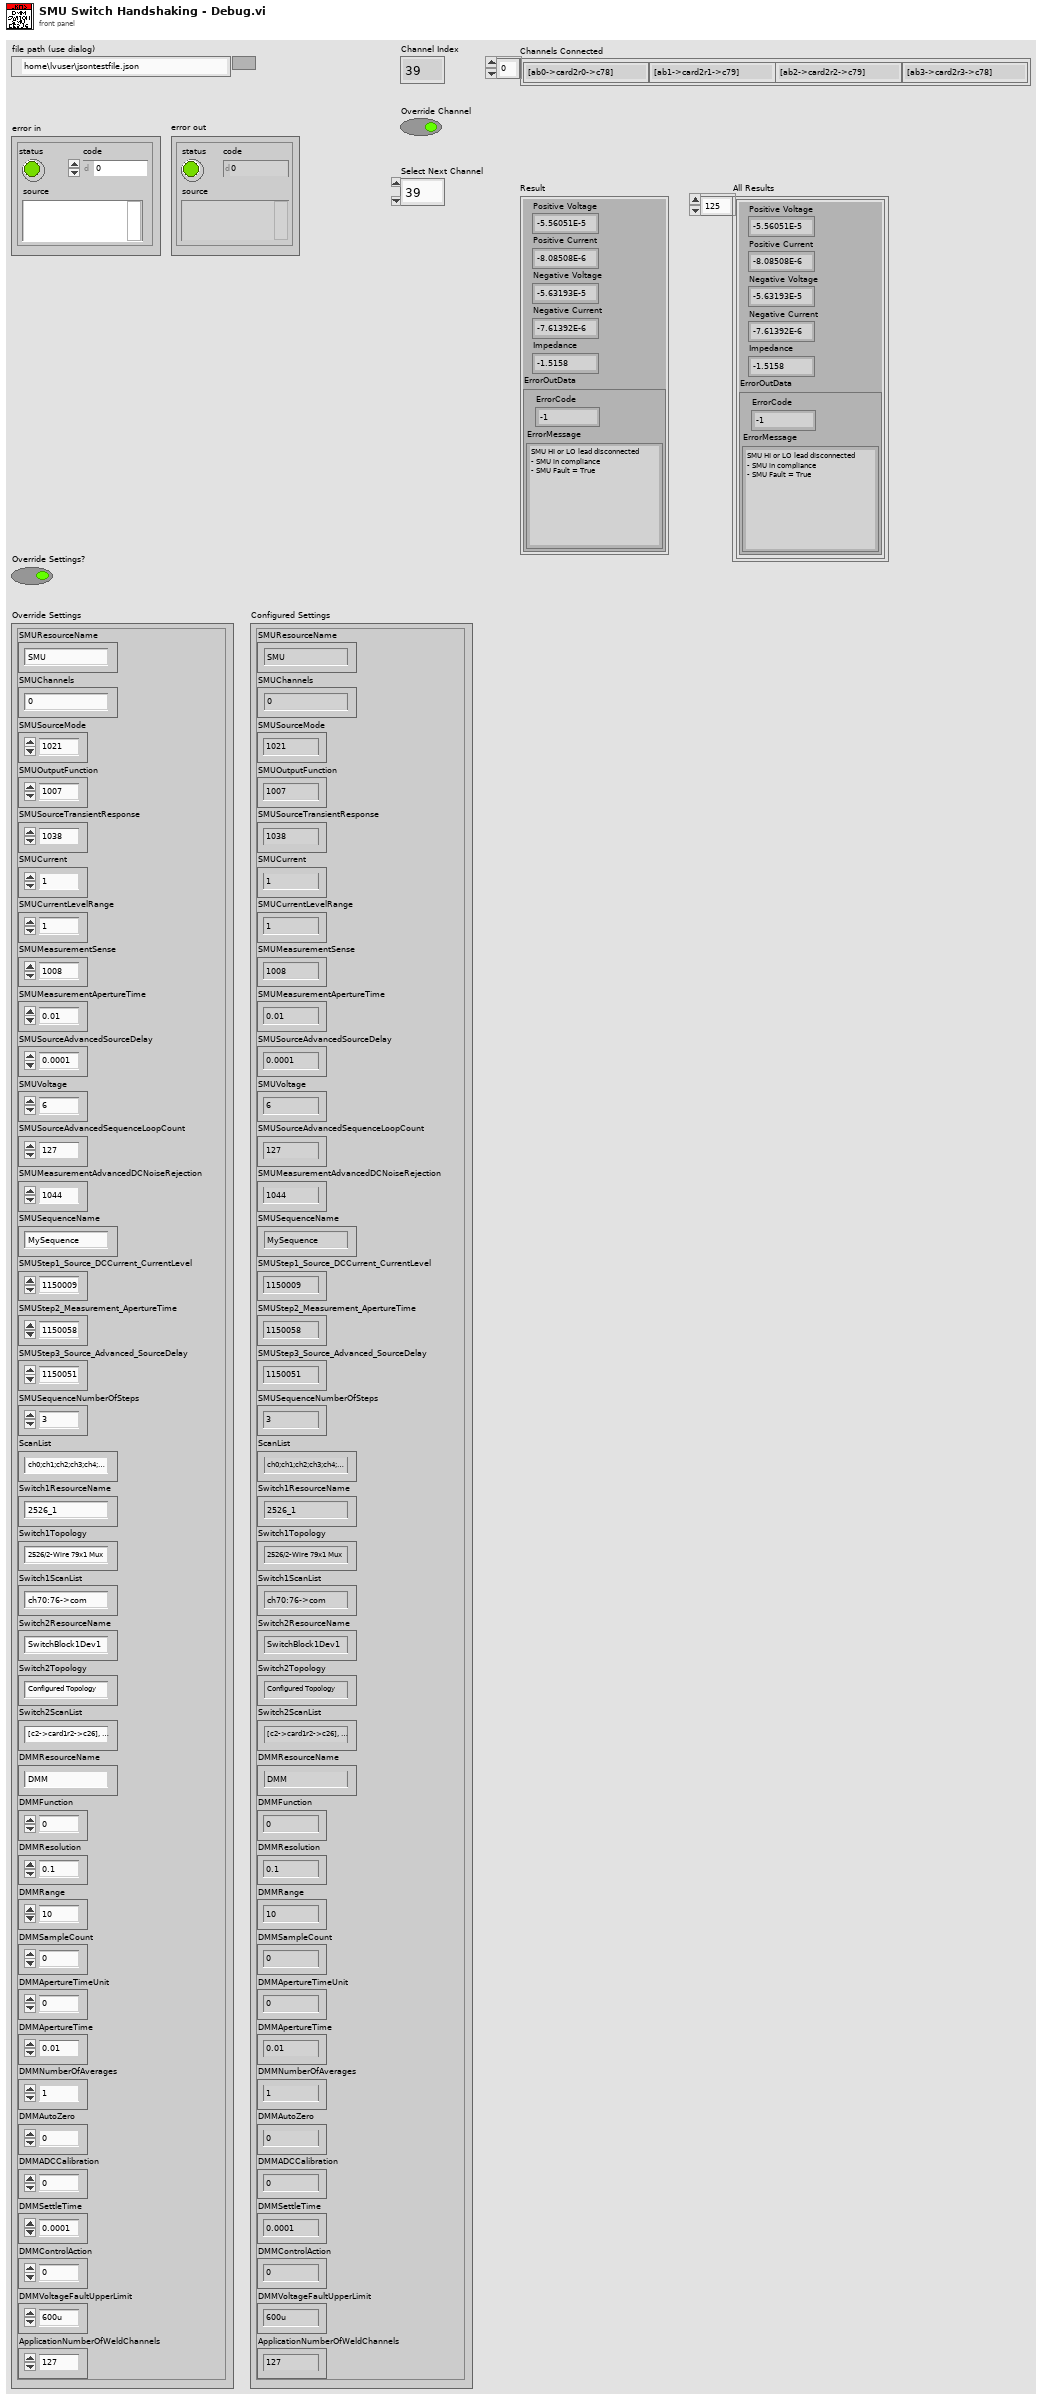
[diagram p1: front panel]
types:
  T1 = typedef "JSONCluster.ctl" = cluster{"SMUResourceName":string, "SMUChannels":string, "SMUSourceMode":i32, "SMUOutputFunction":i32, "SMUSourceTransientResponse":i32, "SMUCurrent":dbl, "SMUCurrentLevelRange":dbl, "SMUMeasurementSense":i32, "SMUMeasurementApertureTime":dbl, "SMUSourceAdvancedSourceDelay":dbl, "SMUVoltage":dbl, "SMUSourceAdvancedSequenceLoopCount":i32, "SMUMeasurementAdvancedDCNoiseRejection":i32, "SMUSequenceName":string, "SMUStep1_Source_DCCurrent_CurrentLevel":i32, "SMUStep2_Measurement_ApertureTime":i32, "SMUStep3_Source_Advanced_SourceDelay":i32, "SMUSequenceNumberOfSteps":i32, "ScanList":string, "Switch1ResourceName":string, "Switch1Topology":string, "Switch1ScanList":string, "Switch2ResourceName":string, "Switch2Topology":string, "Switch2ScanList":string, "DMMResourceName":string, "DMMFunction":i32, "DMMResolution":dbl, "DMMRange":dbl, "DMMSampleCount":i32, "DMMApertureTimeUnit":i32, "DMMApertureTime":dbl, "DMMNumberOfAverages":i32, "DMMAutoZero":i32, "DMMADCCalibration":i32, "DMMSettleTime":dbl, "DMMControlAction":i32, "DMMVoltageFaultUpperLimit":dbl, "ApplicationNumberOfWeldChannels":i32}
  T2 = typedef "labview-grpc-measurement-server.lvlib/MeasurementServer_FourProbeRawData.ctl" = cluster{"Positive Voltage":dbl, "Positive Current":dbl, "Negative Voltage":dbl, "Negative Current":dbl, "Impedance":dbl, "ErrorOutData":T3}
  T3 = typedef "labview-grpc-measurement-server.lvlib/MeasurementServer_ErrorOutData.ctl" = cluster{"ErrorCode":i32, "ErrorMessage":string}
  T4 = typedef "niDCPower Send Software Edge Trigger - Signal.ctl" = i32
  T5 = typedef "niDMM Acquisition State.ctl" = enum16{"Running", "Finished with Backlog", "Finished with no Backlog", "Paused", "No acquisition in progress"}
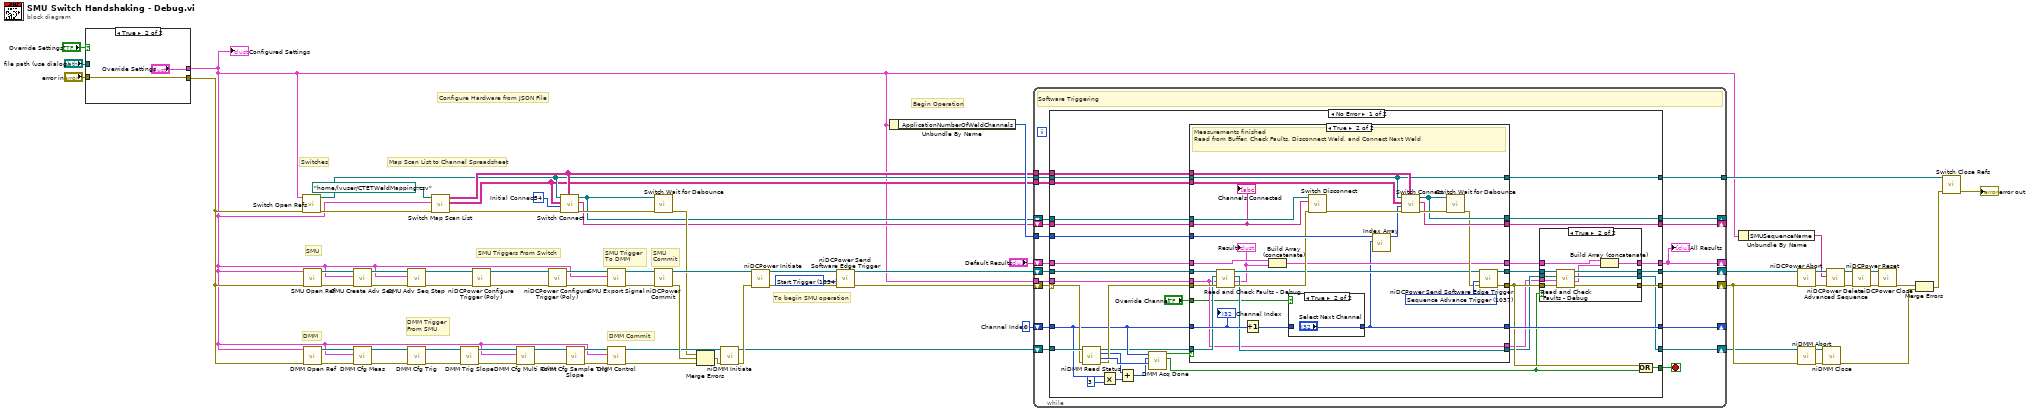
[diagram p0: block diagram]
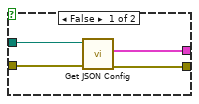
[diagram p2: hidden frame]
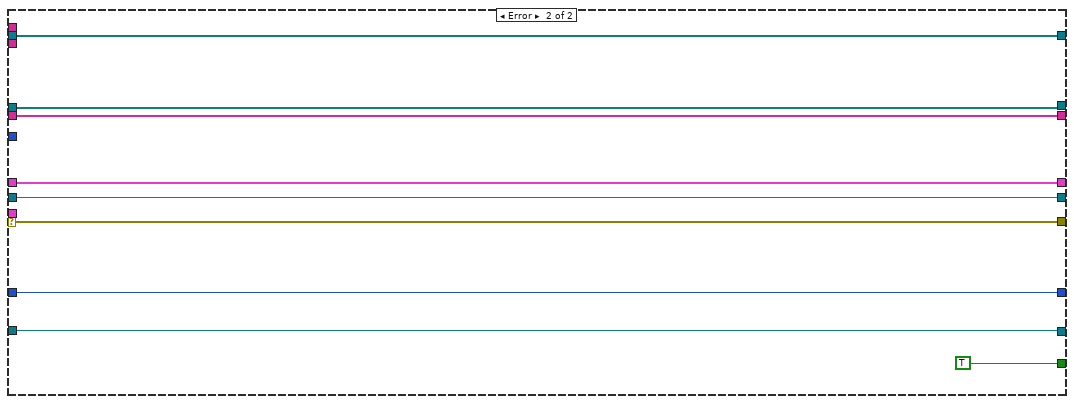
[diagram p6: hidden frame]
diagram:
  w16 = 54  # Initial Connect
  w29 = 0  # Channel Index
  w30 = T4 1034 items=["Start Trigger"=1034, "Source Trigger"=1035, "Measure Trigger"=1036, "Sequence Advance Trigger"=1037, "Pulse Trigger"=1053] ("signal")
  # "Map Scan List to Channel Spreadsheet"
  # "SMU\nCommit"
  # "DMM Commit"
  # "Begin Operation"
  # "Configure Hardware from JSON File"
  # "DMM"
  # "SMU"
  # "Switches"
  # "To begin SMU operation"
  # "DMM Trigger\nFrom SMU"
  # "SMU Trigger \nTo DMM"
  # "SMU Triggers From Switch"
  n1 = case shown="True" "Override Settings?" {
    tunnel: "file path (use dialog)" -> [w76 _]
    tunnel: "error in" -> [w75 w78]
    tunnel: [w74 w78] -> w15
    tunnel: [w73 "Override Settings"] -> w5
    frame False {
      n2 = call "Get JSON Config.vi"("error in (no error)"=w75, "JSON Configuration File (.json)"=w76) -> ("error out"=w74:errorcluster, "JSONCluster"=w73:T1)  [unwired: 6 in, 2 out]
    }
    frame True {
    }
  }
  "Configured Settings" <- w5
  n3 = call "Switch Open Refs.vi"("error in"=w15, "JSONCluster"=w5) -> ("error out"=w19:errorcluster, "Switch Refs"=w12:refnum<k15>[])  [unwired: 8 in]
  n4 = call "SMU Open Ref.vi"("error in (no error)"=w15, "JSONCluster"=w5) -> ("error out"=w71:errorcluster, "IVI Refnum out"=w72:refnum<k15>)  [unwired: 8 in]
  n5 = call "DMM Open Ref.vi"("error in"=w15, "JSONCluster"=w5) -> ("error out"=w46:errorcluster, "IVI Refnum out"=w45:refnum<k15>)  [unwired: 8 in]
  n6 = call "SMU Create Adv Seq.vi"("error in (no error)"=w71, "JSONCluster"=w5, "IVI Refnum in"=w72) -> ("error out"=w61:errorcluster, "IVI Refnum out"=w62:refnum<k15>)  [unwired: 7 in]
  n7 = call "DMM Cfg Meas.vi"("error in (no error)"=w46, "JSONCluster"=w5, "IVI Refnum in"=w45) -> ("error out"=w50:errorcluster, "IVI Refnum out"=w49:refnum<k15>)  [unwired: 7 in]
  n8 = call "SMU Adv Seq Step.vi"("error in (no error)"=w61, "JSONCluster"=w5, "IVI Refnum in"=w62) -> ("error out"=w59:errorcluster, "IVI Refnum out"=w60:refnum<k15>)  [unwired: 7 in]
  n9 = call "DMM Cfg Trig.vi"("error in (no error)"=w50, "IVI Refnum in"=w49) -> ("error out"=w52:errorcluster, "IVI Refnum out"=w51:refnum<k15>)  [unwired: 8 in]
  n10 = call "Switch Map Scan List.vi"("error in (no error)"=w19, "JSONCluster"=w5, "Ch Spreadsheet"=path "/home/lvuser/CTETWeldMapping.csv") -> ("error out"=w18:errorcluster, "IVI Specifications"=w11:string[][], "Channel Specs"=w13:string[][])  [unwired: 6 in]
  n11 = call "DMM Trig Slope.vi"("error in (no error)"=w52, "IVI Refnum in"=w51) -> ("error out"=w54:errorcluster, "IVI Refnum out"=w53:refnum<k15>)  [unwired: 8 in]
  n12 = call-poly <instrlib>:"niDCPower Configure Trigger (Poly).vi"("error in (no error)"=w59, "instrument handle"=w60) -> ("error out"=w69:errorcluster, "instrument handle out"=w70:refnum<k15>)  [unwired: 8 in]
  n13 = call "DMM Cfg Multi Point.vi"("error in (no error)"=w54, "JSONCluster"=w5, "IVI Refnum in"=w53) -> ("error out"=w56:errorcluster, "IVI Refnum out"=w55:refnum<k15>)  [unwired: 7 in]
  n14 = call-poly <instrlib>:"niDCPower Configure Trigger (Poly).vi"("error in (no error)"=w69, "instrument handle"=w70) -> ("error out"=w34:errorcluster, "instrument handle out"=w35:refnum<k15>)  [unwired: 8 in]
  n15 = call "Switch Connect.vi"("Channel Specs"=w13, "error in (no error)"=w18, "Channel Index"=w16, "IVI Specifications"=w11, "Switch Refs"=w12) -> ("error out"=w17:errorcluster, "Channels Connected"=w9:string[], "Refs Connected"=w10:refnum<k15>[])  [unwired: 4 in]
  n16 = call "DMM Cfg Sample Trig Slope.vi"("error in (no error)"=w56, "IVI Refnum in"=w55) -> ("error out"=w38:errorcluster, "IVI Refnum out"=w39:refnum<k15>)  [unwired: 8 in]
  n17 = call "SMU Export Signal.vi"("error in (no error)"=w34, "JSONCluster"=w5, "IVI Refnum in"=w35) -> ("error out"=w57:errorcluster, "IVI Refnum out"=w58:refnum<k15>)  [unwired: 7 in]
  n18 = call "DMM Control.vi"("error in (no error)"=w38, "JSONCluster"=w5, "IVI Refnum in"=w39) -> ("error out"=w43:errorcluster, "IVI Refnum out"=w40:refnum<k15>)  [unwired: 7 in]
  n19 = call "Switch Wait for Debounce.vi"("error in (no error)"=w17, "Switch Refs"=w10) -> ("error out"=w14:errorcluster)  [unwired: 9 in]
  n20 = call <instrlib>:"niDCPower Commit.vi"("error in (no error)"=w57, "instrument handle"=w58) -> ("error out"=w44:errorcluster, "instrument handle out"=w41:refnum<k15>)  [unwired: 8 in]
  n21 = Merge Errors(w14, w44, w43) -> (w42:errorcluster)
  n22 = call <instrlib>:"niDMM Initiate.vi"("error in (no error)"=w42, "instrument handle"=w40) -> ("error out"=w26:errorcluster, "instrument handle out"=w23:refnum<k15>)  [unwired: 8 in]
  n23 = call <instrlib>:"niDCPower Initiate.vi"("error in (no error)"=w26, "instrument handle"=w41) -> ("error out"=w27:errorcluster, "instrument handle out"=w31:refnum<k15>)  [unwired: 8 in]
  n24 = call <instrlib>:"niDCPower Send Software Edge Trigger.vi"("error in (no error)"=w27, "signal"=w30, "instrument handle"=w31) -> ("error out"=w21:errorcluster, "instrument handle out"=w24:refnum<k15>)  [unwired: 7 in]
  n25 = Unbundle By Name(w5) -> ("ApplicationNumberOfWeldChannels"=w28:i32)
  n26 = while {
    shift-right: [w99] -> w4
    shift-left: w24 -> [w98]
    shift-right: [w92] -> w22
    shift-left: w21 -> [w90]
    shift-right: [w94] -> w3
    shift-left: w23 -> [w95]
    shift-right: [w97] -> _
    shift-left: w29 -> [w93]
    tunnel: w28 -> [w96]
    tunnel: w13 -> [w89]
    tunnel: w12 -> [w88]
    tunnel: w11 -> [w87]
    shift-right: [w83] -> _
    shift-left: w10 -> [w86]
    shift-right: [w82] -> _
    shift-left: w9 -> [w85]
    tunnel: [w84] -> w8
    tunnel: w5 -> [w81]
    shift-right: [w79] -> _
    shift-left: "Default Results" -> [w80]
    stop <- w91 stop-if-true
    # "Software Triggering"
    n27 = case shown="No Error" w90 {
      selector: w90 -> [w128 w195]
      tunnel: [w104 w194] -> w99
      tunnel: w98 -> [w135 w194]
      tunnel: [w134 w196] -> w97
      tunnel: w96 -> [w133 _]
      tunnel: w95 -> [w131 w197]
      tunnel: [w102 w197] -> w94
      tunnel: w93 -> [w125 w196]
      tunnel: [w109 w195] -> w92
      tunnel: [w122 TRUE] -> w91
      tunnel: w89 -> [w121 _]
      tunnel: w88 -> [w120 w193]
      tunnel: w87 -> [w119 _]
      tunnel: w86 -> [w118 w192]
      tunnel: w85 -> [w117 w191]
      tunnel: [w116 w193] -> w84
      tunnel: [w115 w192] -> w83
      tunnel: [w114 w191] -> w82
      tunnel: w81 -> [w112 _]
      tunnel: w80 -> [w111 w190]
      tunnel: [w107 w190] -> w79
      frame No Error {
        n28 = call <instrlib>:"niDMM Read Status.vi"("error in (no error)"=w128, "instrument handle"=w131) -> ("error out"=w130:errorcluster, "Acquisition State"=w132:T5, "Backlog"=w127:i32, "instrument handle out"=w113:refnum<k15>)  [unwired: 6 in]
        n29 = Multiply(x=w125, y=3) -> (x*y=w123:i32)
        n30 = Add(x=w127, y=w123) -> (x+y=w126:i32)
        n31 = call "DMM Acq Done.vi"("Acquisition State"=w132, "Backlog"=w126, "Channel Index"=w125) -> ("Finished with Backlog?"=w106:bool, "Sequence Acquision Finished?"=w129:bool)  [unwired: 7 in]
        n32 = case shown="True" w129 {
          tunnel: w130 -> [w157 w170]
          tunnel: [w158 w187] -> w105
          tunnel: [w157 w186] -> w110
          tunnel: w135 -> [w158 w171]
          tunnel: w125 -> [w156 w184]
          tunnel: [w156 w160] -> w134
          tunnel: w133 -> [_ w183]
          tunnel: w121 -> [_ w180]
          tunnel: w120 -> [w155 w175]
          tunnel: w119 -> [_ w179]
          tunnel: w118 -> [w154 w178]
          tunnel: w117 -> [w153 w177]
          tunnel: [w155 w175] -> w116
          tunnel: [w154 w174] -> w115
          tunnel: [w153 w173] -> w114
          tunnel: w113 -> [w152 w167]
          tunnel: [w152 w166] -> w103
          tunnel: w112 -> [w150 w164]
          tunnel: w111 -> [w151 w163]
          tunnel: [w151 w165] -> w108
          tunnel: [w150 w164] -> w101
          tunnel: "Override Channel" -> [_ w159]
          frame False {
            # "Measurements not finished yet - repeat loop"
          }
          frame True {
            w185 = T4 1037 items=["Start Trigger"=1034, "Source Trigger"=1035, "Measure Trigger"=1036, "Sequence Advance Trigger"=1037, "Pulse Trigger"=1053] ("signal")
            # "Measurements finished\nRead from Buffer, Check Faults, Disconnect Weld, and Connect Next Weld"
            n33 = call "Read and Check Faults - Debug.vi"("error in (no error)"=w170, "JSONCluster"=w164, "DMM Ref"=w167, "SMU Ref"=w171) -> ("error out"=w169:errorcluster, "Result"=w162:T2, "DMM Ref Out"=w166:refnum<k15>, "SMU Ref Out"=w168:refnum<k15>)  [unwired: 4 in]
            "Result" <- w162
            n34 = Increment(x=w184) -> (x+1=w161:i32)
            n35 = Build Array (concatenate)(w163, w162) -> (w165:T2[])
            n36 = case shown="True" w159 {
              tunnel: w161 -> [w188 _]
              tunnel: [w188 "Select Next Channel"] -> w160
              frame False {
              }
              frame True {
              }
            }
            n37 = call "Switch Disconnect.vi"("error in (no error)"=w169, "Channels Connected"=w177, "Switch Refs"=w178) -> ("error out"=w182:errorcluster)  [unwired: 8 in]
            n38 = call "Index Array.vi"("Backlog"=w160, "ApplicationNumberOfWeldChannels"=w183) -> ("Index"=w176:i32)  [unwired: 9 in]
            n39 = call "Switch Connect.vi"("Channel Specs"=w180, "error in (no error)"=w182, "Channel Index"=w176, "IVI Specifications"=w179, "Switch Refs"=w175) -> ("error out"=w181:errorcluster, "Channels Connected"=w173:string[], "Refs Connected"=w174:refnum<k15>[])  [unwired: 4 in]
            n40 = call "Switch Wait for Debounce.vi"("error in (no error)"=w181, "Switch Refs"=w174) -> ("error out"=w172:errorcluster)  [unwired: 9 in]
            n41 = call <instrlib>:"niDCPower Send Software Edge Trigger.vi"("error in (no error)"=w172, "signal"=w185, "instrument handle"=w168) -> ("error out"=w186:errorcluster, "instrument handle out"=w187:refnum<k15>)  [unwired: 7 in]
            "Channel Index" <- w184
            "Channels Connected" <- w177
          }
        }
        n42 = case shown="True" w106 {
          tunnel: w110 -> [w137 w149]
          tunnel: [w137 w148] -> w109
          tunnel: w108 -> [w139 w141]
          tunnel: [w139 w147] -> w107
          tunnel: w105 -> [w138 w146]
          tunnel: [w138 w145] -> w104
          tunnel: w103 -> [w136 w144]
          tunnel: [w136 w143] -> w102
          tunnel: w101 -> [_ w142]
          frame False {
          }
          frame True {
            n43 = call "Read and Check Faults - Debug.vi"("error in (no error)"=w149, "JSONCluster"=w142, "DMM Ref"=w144, "SMU Ref"=w146) -> ("error out"=w148:errorcluster, "Result"=w140:T2, "DMM Ref Out"=w143:refnum<k15>, "SMU Ref Out"=w145:refnum<k15>)  [unwired: 4 in]
            n44 = Build Array (concatenate)(w141, w140) -> (w147:T2[])
          }
        }
        n45 = Compound Arithmetic op=OR(w110, w106) -> (w122:bool)
      }
      frame Error {
      }
    }
    "All Results" <- w79
  }
  n46 = Unbundle By Name(w5) -> ("SMUSequenceName"=w25:string)
  n47 = call <instrlib>:"niDCPower Abort.vi"("error in (no error)"=w22, "instrument handle"=w4) -> ("error out"=w67:errorcluster, "instrument handle out"=w68:refnum<k15>)  [unwired: 8 in]
  n48 = call <instrlib>:"niDMM Abort.vi"("error in (no error)"=w22, "instrument handle"=w3) -> ("error out"=w48:errorcluster, "instrument handle out"=w47:refnum<k15>)  [unwired: 8 in]
  n49 = call <instrlib>:"niDMM Close.vi"("error in (no error)"=w48, "instrument handle"=w47) -> ("error out"=w37:errorcluster)  [unwired: 9 in]
  n50 = call <instrlib>:"niDCPower Delete Advanced Sequence.vi"("error in (no error)"=w67, "sequence name"=w25, "instrument handle"=w68) -> ("error out"=w66:errorcluster, "instrument handle out"=w65:refnum<k15>)  [unwired: 7 in]
  n51 = call <instrlib>:"niDCPower Reset.vi"("error in (no error)"=w66, "instrument handle"=w65) -> ("error out"=w63:errorcluster, "instrument handle out"=w64:refnum<k15>)  [unwired: 2 in, 6 out]
  n52 = call <instrlib>:"niDCPower Close.vi"("error in (no error)"=w63, "instrument handle"=w64) -> ("error out"=w36:errorcluster)  [unwired: 9 in]
  n53 = Merge Errors(w36, w37) -> (w7:errorcluster)
  n54 = call "Switch Close Refs.vi"("error in (no error)"=w7, "Switch Refs"=w8) -> ("error out"=→"error out":errorcluster)  [unwired: 9 in]
